vi "simple_chat_bot.vi"() -> ()   [LabVIEW 2020]
uses:
  <userlib>/_Soliton/LabVIEW LLM Libraries/models/message_text/message_text.lvclass
  C:/Program Files/National Instruments/LabVIEW 2020/user.lib/_Soliton/LabVIEW LLM Libraries/models/abstract_message_base/abstract_message_base.lvclass
  <userlib>/_Soliton/LabVIEW LLM Libraries/models/llm_openai_chatmodels/llm_openai_chatmodels.lvclass
  C:/Program Files/National Instruments/LabVIEW 2020/user.lib/_Soliton/LabVIEW LLM Libraries/models/abstract_llm_base/abstract_llm_base.lvclass
  <userlib>/_Soliton/LabVIEW LLM Libraries/models/llm_openai_chatmodels/Instantiate_llm_openai.vi
  <userlib>/_Soliton/LabVIEW LLM Libraries/models/message_text/create_text_message.vi
  <userlib>/_Soliton/LabVIEW LLM Libraries/user_interfaces/simple_html_chat_ui/simple_html_chat_ui.lvclass
  <userlib>/_Soliton/LabVIEW LLM Libraries/models/abstract_llm_chatcompletion/abstract_llm_chatcompletion.lvclass
panel:
  in  "new_message":string
  in  "send":bool
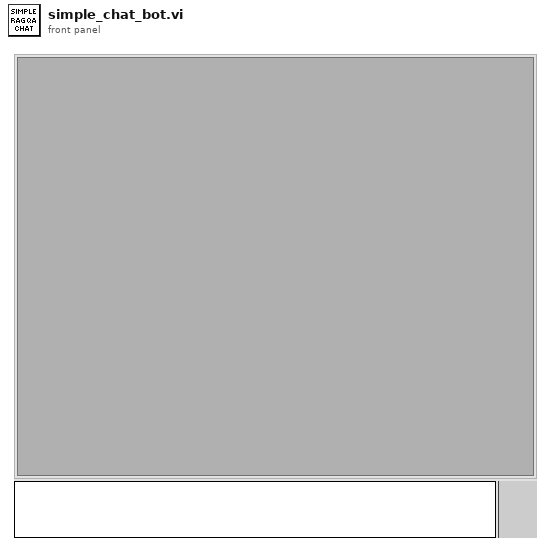
[diagram p1: front panel]
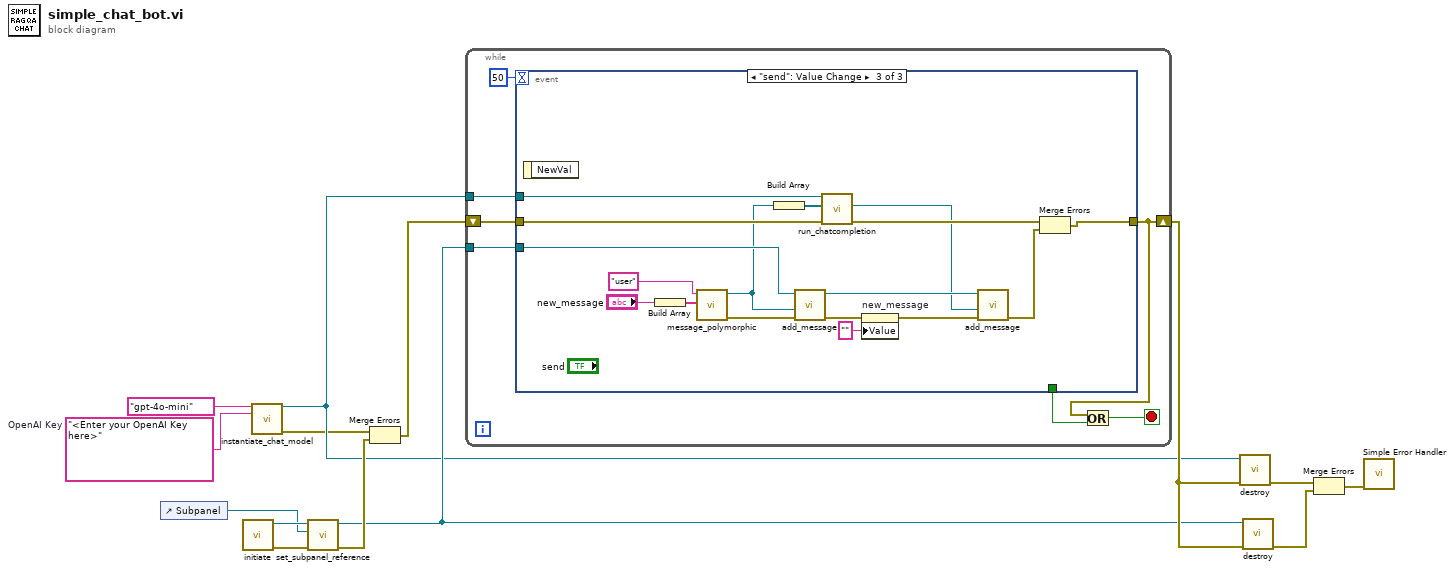
[diagram p0: block diagram]
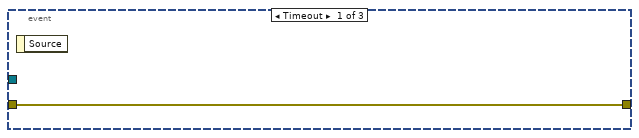
[diagram p2: hidden frame]
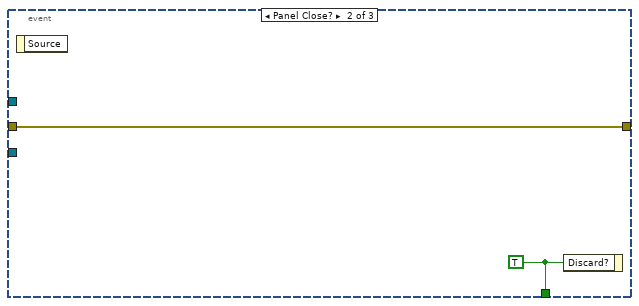
[diagram p3: hidden frame]
diagram:
  w4 = "<Enter your OpenAI Key here>"  # OpenAI Key
  n1 = control-ref of="Subpanel"() -> (w8:refnum<vi>)
  n2 = call <userlib>:"initiate.vi"() -> ("error out"=w11:errorcluster, "simple_html_chat_ui out"=w9:refnum<class "simple_html_chat_ui.lvclass">)  [unwired: 10 in]
  n3 = call-poly <userlib>:"instantiate_chat_model.vi"("model_name"="gpt-4o-mini", "openai_key"=w4) -> ("llm_openai out"=w3:refnum<class "llm_openai_chatmodels.lvclass">, "error out"=w1:errorcluster)  [unwired: 12 in]
  n4 = call <userlib>:"set_subpanel_reference.vi"("error in (no error)"=w11, "Sub Panel"=w8, "simple_html_chat_ui in"=w9) -> ("error out"=w10:errorcluster, "simple_html_chat_ui out"=w5:refnum<class "simple_html_chat_ui.lvclass">)  [unwired: 7 in]
  n5 = Merge Errors(w1, w10) -> (w12:errorcluster)
  n6 = while {
    shift-right: [w17] -> w7
    shift-left: w12 -> [w19]
    tunnel: w5 -> [w16]
    tunnel: w3 -> [w15]
    stop <- w18 stop-if-true
    n7 = event shown="[2] \"send\": Value Change" {
      selector: _ -> [_ _ _]
      dyn-events: _ -> [_ _ _]
      timeout: 50 -> [_ _ _]
      tunnel: [_ w24 _] -> w21
      tunnel: w19 -> [w22 w23 w29]
      tunnel: [w22 w23 w38] -> w17
      tunnel: w16 -> [_ _ w35]
      tunnel: w15 -> [_ _ w26]
      event Timeout {
        n8 = event-data() -> ()  [unwired: 1 in, 1 out]
      }
      event Panel Close? {
        w24 = TRUE ("Discard?")
        n9 = event-data() -> ()  [unwired: 1 in, 1 out]
        n10 = event-data("Discard?"=w24) -> ()  [unwired: 1 in, 1 out]
      }
      event "send": Value Change {
        n11 = event-data() -> ()  [unwired: 1 in, 1 out]
        n12 = Build Array("new_message") -> (w39:string[])
        n13 = call-poly <userlib>:"message_polymorphic.vi"("content"=w39, "role"="user") -> ("error out"=w36:errorcluster, "message_text out"=w28:refnum<class "message_text.lvclass">)  [unwired: 8 in]
        n14 = Build Array(w28) -> (w27:refnum<class "message_text.lvclass">[])
        n15 = call <userlib>:"add_message.vi"("error in (no error)"=w36, "Message"=w28, "simple_html_chat_ui in"=w35) -> ("error out"=w33:errorcluster, "simple_html_chat_ui out"=w34:refnum<class "simple_html_chat_ui.lvclass">)  [unwired: 7 in]
        n16 = call <userlib>:"run_chatcompletion.vi"("error in (no error)"=w29, "Messages"=w27, "abstract_llm_chatcompletion in"=w26) -> ("error out"=w30:errorcluster, "Response"=w25:refnum<class "abstract_message_base.lvclass">)  [unwired: 6 in, 1 out]
        n17 = property on="new_message" class="Str"(error in=w33, "Value"="" ("new_message")) -> (error out=w32:errorcluster)  [unwired: 1 in, 1 out]
        n18 = call <userlib>:"add_message.vi"("error in (no error)"=w32, "Message"=w25, "simple_html_chat_ui in"=w34) -> ("error out"=w37:errorcluster)  [unwired: 7 in, 1 out]
        n19 = Merge Errors(w30, w37) -> (w38:errorcluster)
      }
    }
    n20 = Or(x=w17, y=w21) -> (x .or. y?=w18:bool)
  }
  n21 = call-dynamic <userlib>:"destroy.vi"("error in (no error)"=w7, "abstract_llm_base in"=w3) -> ("error out"=w2:errorcluster)  [unwired: 8 in, 1 out]
  n22 = call <userlib>:"destroy.vi"("error in (no error)"=w7, "simple_html_chat_ui in"=w5) -> ("error out"=w6:errorcluster)  [unwired: 8 in, 1 out]
  n23 = Merge Errors(w2, w6) -> (w13:errorcluster)
  n24 = call <vilib>:"Simple Error Handler.vi"("error in (no error)"=w13) -> ()  [unwired: 4 in, 5 out]
